vi "DAC_send_order.vi"(4 "secured?":bool, 6 "DAC goto value":sgl, 7 "order":T2(ring)=enum."buses to use", 8 "Cluster":cluster{"panel":u8, "channel":u8}, 9 "delay between steps (ms)":u8, 10 "buses to use":bool[](array[boolean]), 11 "FPGA VI Reference In":T1) -> (3 "FPGA VI Reference Out":T1)   [LabVIEW 2013]
uses:
  fpga-bitfile-ref.ctl
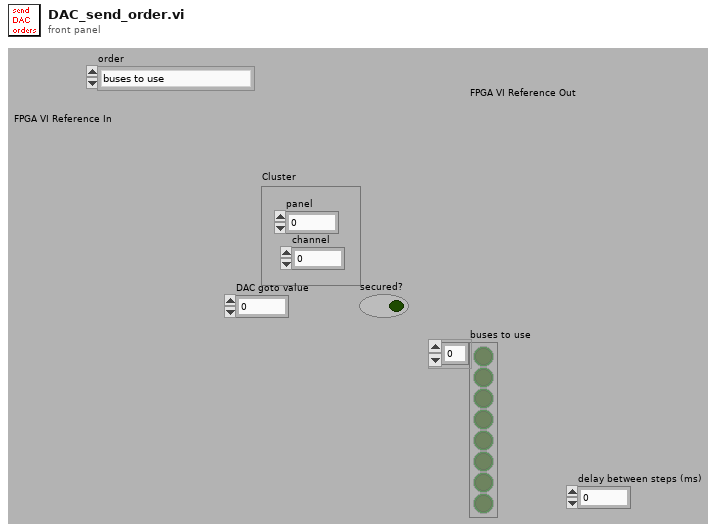
[diagram p1: front panel]
types:
  T1 = typedef "fpga-bitfile-ref.ctl" = refnum<k20>
  T2 = enum8{"start movement", "buses to use", "delay", "value", "stop", ""}
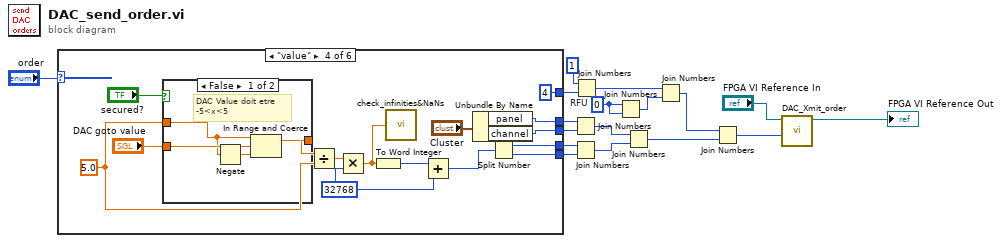
[diagram p0: block diagram]
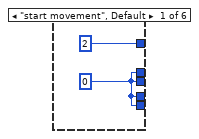
[diagram p2: hidden frame]
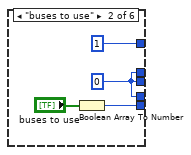
[diagram p3: hidden frame]
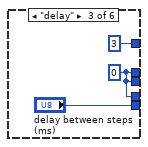
[diagram p4: hidden frame]
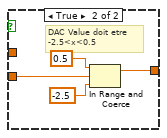
[diagram p5: hidden frame]
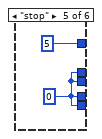
[diagram p6: hidden frame]
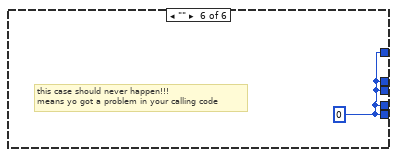
[diagram p7: hidden frame]
diagram:
  w17 = u8 0  # RFU
  n1 = case shown="\"value\"" "order" {
    tunnel: [w19 w23 w25 w41 w50 w52] -> w13
    tunnel: [w19 w23 w25 w37 w50 w52] -> w15
    tunnel: [w19 w23 w25 w36 w50 w52] -> w16
    tunnel: [w19 w21 "delay between steps (ms)" w40 w50 w52] -> w14
    tunnel: [u8 2 ("order") u8 1 ("order") u8 3 ("order") u8 4 ("order") u8 5 ("delay between steps (ms)") w52] -> w4
    frame "start movement", Default {
      w19 = u8 0
    }
    frame "buses to use" {
      w23 = u8 0
      n2 = Boolean Array To Number(Boolean array="buses to use") -> (number=w21:u8)
    }
    frame "delay" {
      w25 = u8 0 ("RFU")
    }
    frame "value" {
      w27 = 5.0 ("Double")
      w33 = u16 32768 ("y")
      n3 = case shown="False" "secured?" {
        tunnel: "DAC goto value" -> [w45 w49]
        tunnel: [w44 w48] -> w31
        tunnel: w27 -> [w43 _]
        frame False {
          # "DAC Value doit etre\n-5<x<5"
          n4 = Negate(x=w43) -> (-x=w42:dbl)
          n5 = In Range and Coerce(upper limit=w43, x=w45, lower limit=w42) -> (coerced(x)=w44:dbl)  [unwired: 1 out]
        }
        frame True {
          # "DAC Value doit etre\n-2.5<x<0.5"
          n6 = In Range and Coerce(upper limit=sgl 0.5, x=w49, lower limit=sgl -2.5) -> (coerced(x)=w48:sgl)  [unwired: 1 out]
        }
      }
      n7 = Divide(x=w31, y=w27) -> (x/y=w35:dbl)
      n8 = Multiply(x=w35, y=w33) -> (x*y=w28:dbl)
      n9 = To Word Integer(number=w28) -> (16bit integer=w34:i16)
      n10 = call "check_infinities&NaNs.vi"("Value"=w28) -> ()
      n11 = Add(x=w34, y=w33) -> (x+y=w29:u16)
      n12 = Unbundle By Name("Cluster") -> ("panel"=w36:u8, "channel"=w37:u8)
      n13 = Split Number(x=w29) -> (hi(x)=w41:u8, lo(x)=w40:u8)
    }
    frame "stop" {
      w50 = u8 0 ("RFU")
    }
    frame "" {
      w52 = u8 0 ("delay between steps (ms)")
      # "this case should never happen!!!\nmeans yo got a problem in your calling code"
    }
  }
  n14 = Join Numbers(hi=w16, lo=w15) -> ((hi.lo)=w11:u16)
  n15 = Join Numbers(hi=w13, lo=w14) -> ((hi.lo)=w12:u16)
  n16 = Join Numbers(hi=u8 1, lo=w4) -> ((hi.lo)=w9:u16)
  n17 = Join Numbers(hi=w17, lo=w17) -> ((hi.lo)=w10:u16)
  n18 = Join Numbers(hi=w11, lo=w12) -> ((hi.lo)=w7:u32)
  n19 = Join Numbers(hi=w9, lo=w10) -> ((hi.lo)=w6:u32)
  n20 = Join Numbers(hi=w6, lo=w7) -> ((hi.lo)=w3:u64)
  n21 = call "DAC_Xmit_order.vi"("Order in"=w3, "FPGA VI Reference In"="FPGA VI Reference In") -> ("FPGA VI Reference Out"=→"FPGA VI Reference Out":T1)  [unwired: 9 out]
